vi "Initialize.vi"(8 "error in":errorcluster, 11 "tCRDS Subj in":refnum<class "tCRDS Subj.lvclass">) -> (0 "error out":errorcluster, 2 "DVR":refnum<data-value>, 3 "tCRDS Subj out":refnum<class "tCRDS Subj.lvclass">)   [LabVIEW 2015, in "tCRDS Subj.lvclass"]
doc: "Provides a reference for the CRD Data object."
uses:
  tCRDS Subj.lvclass
  Reusable/Data/Data.lvclass
  CRD/Data/tCRD Data.lvclass
  Reusable/Observer/Data Subject.lvclass/Data Subject.ctl
  Reusable/Observer/Data Subject.lvclass
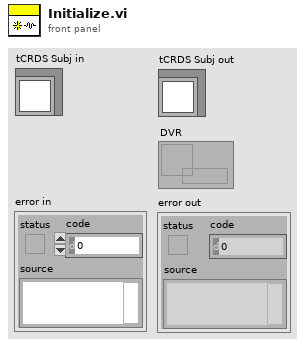
[diagram p1: front panel]
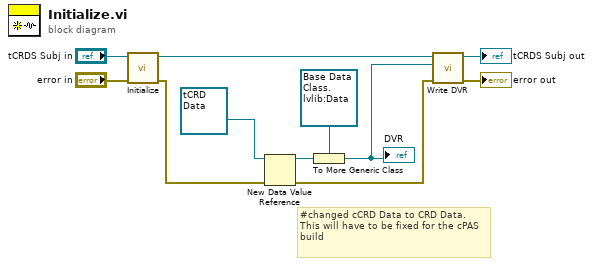
[diagram p0: block diagram]
diagram:
  # "#changed cCRD Data to CRD Data.  This will have to be fixed for the cPAS build"
  n1 = call-parent "Initialize.vi"("error in"="error in", "Data Subject in"="tCRDS Subj in") -> ("error out"=w3:errorcluster, "Data Subject out"=w5:refnum<class "tCRDS Subj.lvclass">)  [unwired: 7 in, 1 out]
  n2 = New Data Value Reference(data value=refnum<class "tCRD Data.lvclass"> refnum ("tCRD Data"), error in=w3) -> (data value reference=w8:refnum<data-value>, error out=w7:errorcluster)
  n3 = To More Generic Class(target class=refnum<data-value> refnum ("data value reference"), reference=w8) -> (generic class reference=w4:refnum<data-value>)
  "DVR" <- w4
  n4 = call "Write DVR.vi"("error in"=w7, "DVR"=w4, "Data Subject in"=w5) -> ("error out"=→"error out":errorcluster, "Data Subject out"=→"tCRDS Subj out":refnum<class "tCRDS Subj.lvclass">)  [unwired: 7 in]
